vi "PushingState.vi"(8 "error in (no error)":errorcluster, 9 "Cluster in":T2, 10 "Enum in":T1, 11 "Actual Start [i]":i64) -> (0 "error out":errorcluster, 2 "Cluster out":T2, 3 "Enum":T1)   [LabVIEW 2018]
uses:
  Type_Def/Type_Def Actuator Controls.ctl
  Type_Def/Type_Def ControlState.ctl
panel:
  out "x-y":dbl
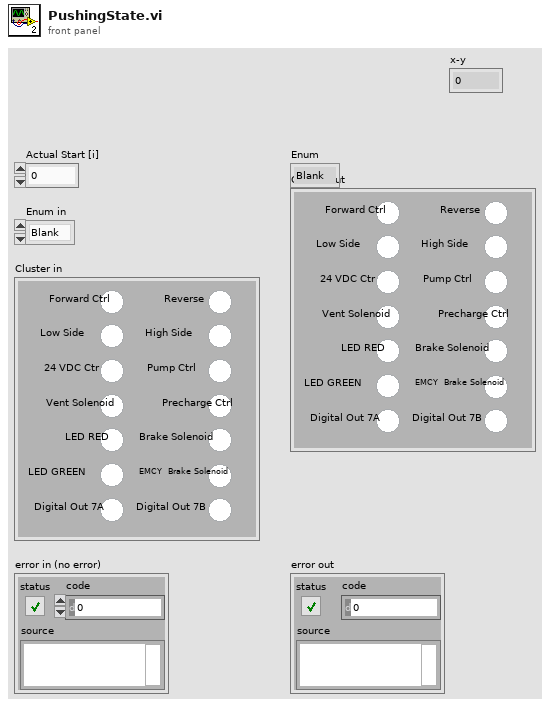
[diagram p1: front panel]
types:
  T1 = typedef "Type_Def ControlState.ctl" = enum16{"Blank", "Systems Check", "Idle", "Ready", "Pushing", "CrawlingPrecharge", "Braking", "Fault", "Boot Up", "Crawling", "Shutdown", "Service Push", "Service Wait", "Vent", "Precharge"}
  T2 = typedef "Type_Def Actuator Controls.ctl" = cluster{"Reverse ":bool, "Precharge Ctrl":bool, "Pump Ctrl":bool, "24 VDC Ctr":bool, "Vent Solenoid":bool, "Brake Solenoid":bool, "EMCY  Brake Solenoid":bool, "Digital Out 7B ":bool, "Forward Ctrl":bool, " Low Side":bool, "High Side":bool, "LED RED":bool, "LED GREEN":bool, " Digital Out 7A":bool}
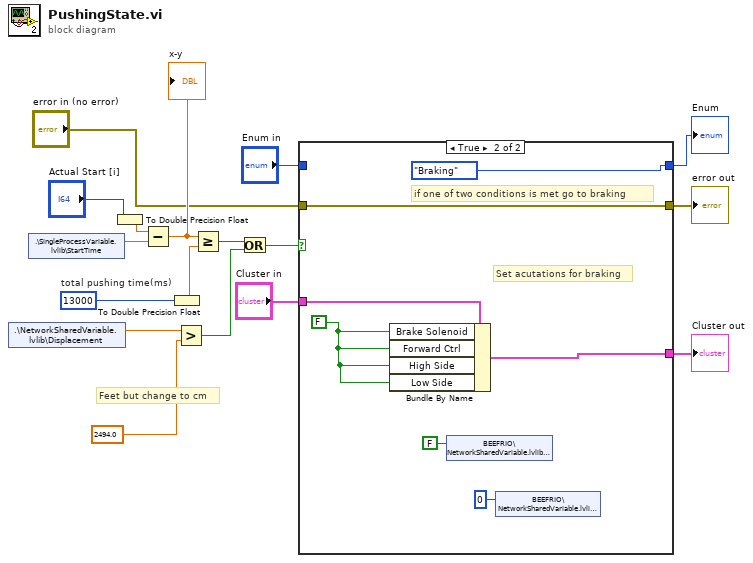
[diagram p0: block diagram]
diagram:
  w12 = i64 13000  # total pushing time(ms)
  # "Feet but change to cm"
  n1 = shared-variable ".\\NetworkSharedVariable.lvlib\\Displacement"() -> (w17:dbl)  [unwired: 1 in, 1 out]
  n2 = shared-variable ".\\SingleProcessVariable.lvlib\\StartTime"() -> (w10:dbl)  [unwired: 1 in, 1 out]
  n3 = To Double Precision Float(number="Actual Start [i]") -> (double precision float=w2:dbl)
  n4 = Subtract(x=w2, y=w10) -> (x-y=w11:dbl)
  "x-y" <- w11
  n5 = To Double Precision Float(number=w12) -> (double precision float=w1:dbl)
  n6 = Greater?(x=w17, y=2494.0 ("Feet but change to cm")) -> (0:w16:bool)
  n7 = Greater Or Equal?(x=w11, y=w1) -> (x >= y?=w13:bool)
  n8 = Or(x=w13, y=w16) -> (x .or. y?=w14:bool)
  n9 = case shown="True" w14 {
    tunnel: "Enum in" -> [w20 _]
    tunnel: [w20 Type_Def_ControlState."Braking"] -> w4
    tunnel: "Cluster in" -> [w19 w26]
    tunnel: [w19 w25] -> w6
    tunnel: [w18 w24] -> w7
    tunnel: "error in (no error)" -> [w18 w24]
    frame False {
      # "If condititon are not meet, then stay  in pushing"
    }
    frame True {
      w23 = FALSE ("Digital Out 5")
      # "Set acutations for braking"
      # "if one of two conditions is met go to braking"
      n10 = Bundle By Name(cluster=w26, "Brake Solenoid"=w23, "Forward Ctrl"=w23, "High Side"=w23, "Low Side"=w23) -> (w25:T2)
      n11 = shared-variable "BEEFRIO\\NetworkSharedVariable.lvlib\\driveEnable"(FALSE ("driveEnable")) -> ()  [unwired: 1 in, 1 out]
      n12 = shared-variable "BEEFRIO\\NetworkSharedVariable.lvlib\\driveTarget"(i16 0 ("driveTarget")) -> ()  [unwired: 1 in, 1 out]
    }
  }
  "error out" <- w7
  "Cluster out" <- w6
  "Enum" <- w4
